vi "Write SQL Ref.vi"(8 "error in (no error)":errorcluster, 10 "connection reference":T1, 11 "Access in":refnum<class "Access.lvclass">) -> (0 "error out":errorcluster, 3 "Access out":refnum<class "Access.lvclass">)   [LabVIEW 2021, in "Database.lvlib" / "Access.lvclass"]
uses:
  Access.lvclass
  <vilib>/addons/database/Connection.llb/Conn ObjectReference.ctl
  Access.lvclass/Access.ctl
  <vilib>/addons/database/NI_Database_API.lvlib
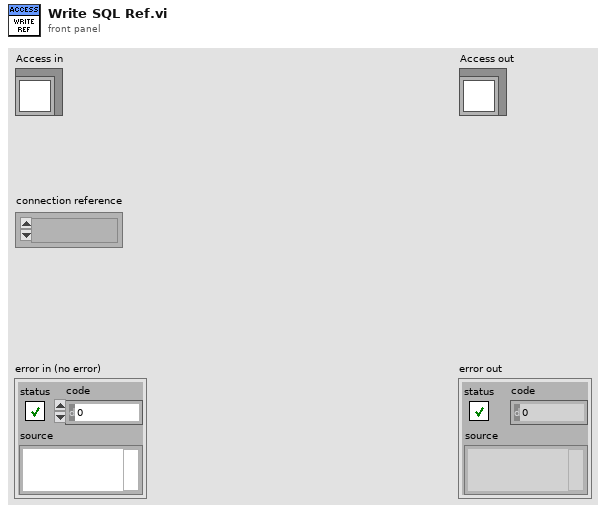
[diagram p1: front panel]
types:
  T1 = typedef "NI_Database_API.lvlib/Conn ObjectReference.ctl" = refnum<k1>
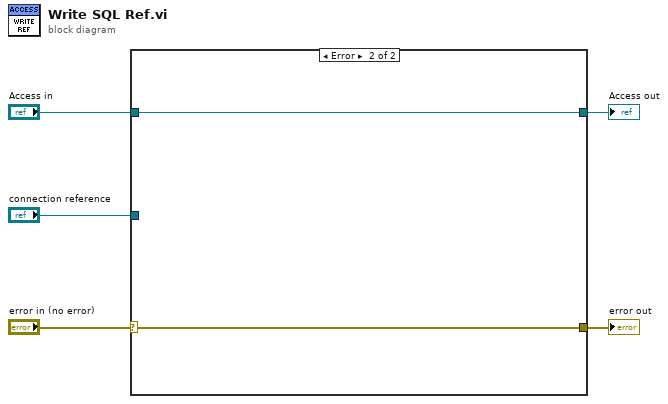
[diagram p0: block diagram]
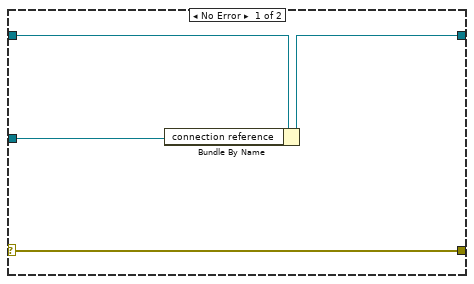
[diagram p2: hidden frame]
diagram:
  n1 = case shown="Error" "error in (no error)" {
    selector: "error in (no error)" -> [w8 w10]
    tunnel: "Access in" -> [w9 w11]
    tunnel: [w7 w11] -> w3
    tunnel: [w8 w10] -> w2
    tunnel: "connection reference" -> [w6 _]
    frame No Error {
      n2 = Bundle By Name(cluster=w9, "connection reference"=w6) -> (w7:refnum<class "Access.lvclass">)
    }
    frame Error {
    }
  }
  "error out" <- w2
  "Access out" <- w3
